vi "Global 1.vi"() -> ()   [LabVIEW 2015]
panel:
  in  "area":dbl
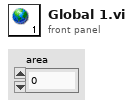
[diagram p1: front panel]
diagram:
